vi "3_HelloAliceBob.vi"() -> ()   [LabVIEW 2015]
panel:
  out "Greeting":string
  in  "Enter your name":string
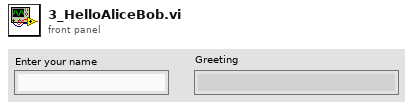
[diagram p1: front panel]
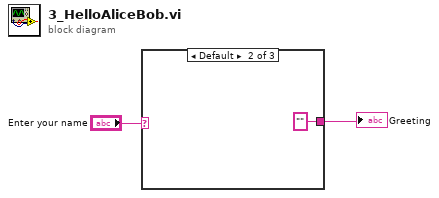
[diagram p0: block diagram]
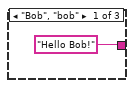
[diagram p2: hidden frame]
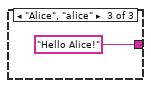
[diagram p3: hidden frame]
diagram:
  n1 = case shown="Default" "Enter your name" {
    tunnel: ["Hello Bob!" "" "Hello Alice!"] -> w1
    frame "Bob", "bob" {
    }
    frame Default {
    }
    frame "Alice", "alice" {
    }
  }
  "Greeting" <- w1
